vi "scaleEncoder.vi"(8 "error in (no error)":errorcluster, 11 "String":string) -> (0 "error out":errorcluster, 2 "Encoder1":i32, 3 "Encoder0":i32)   [LabVIEW 2017]
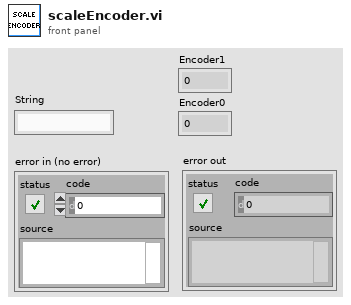
[diagram p1: front panel]
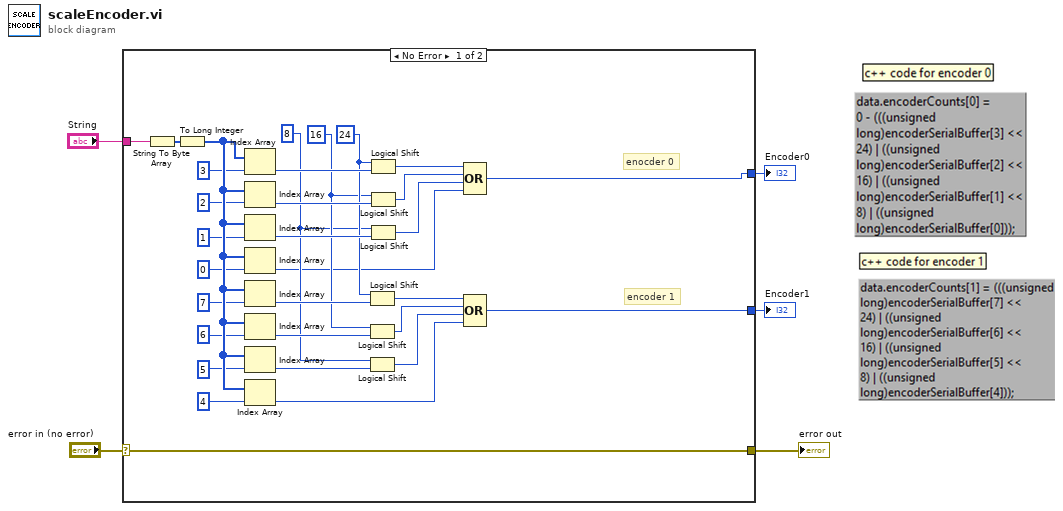
[diagram p0: block diagram]
diagram:
  n1 = case shown="No Error" "error in (no error)" {
    selector: "error in (no error)" -> [w25 w37]
    tunnel: "String" -> [w36 _]
    tunnel: [w25 w37] -> w3
    tunnel: [w7 _] -> w2
    tunnel: [w6 _] -> w1
    frame No Error {
      w16 = 8
      w17 = 16
      w18 = 24
      # "encoder 1"
      # "enocder 0"
      n2 = String To Byte Array(string=w36) -> (unsigned byte array=w35:u8[])
      n3 = To Long Integer(number=w35) -> (32bit integer=w34:i32[])
      n4 = Index Array(array=w34, index=3) -> (element=w24:i32)
      n5 = Index Array(array=w34, index=2) -> (element=w23:i32)
      n6 = Index Array(array=w34, index=1) -> (element=w22:i32)
      n7 = Index Array(array=w34, index=0) -> (element=w12:i32)
      n8 = Index Array(array=w34, index=7) -> (element=w21:i32)
      n9 = Index Array(array=w34, index=6) -> (element=w20:i32)
      n10 = Index Array(array=w34, index=5) -> (element=w19:i32)
      n11 = Index Array(array=w34, index=4) -> (element=w8:i32)
      n12 = Logical Shift(y=w18, x=w21) -> (x << y=w11:i32)
      n13 = Logical Shift(y=w17, x=w20) -> (x << y=w10:i32)
      n14 = Logical Shift(y=w16, x=w19) -> (x << y=w9:i32)
      n15 = Logical Shift(y=w18, x=w24) -> (x << y=w15:i32)
      n16 = Logical Shift(y=w17, x=w23) -> (x << y=w14:i32)
      n17 = Logical Shift(y=w16, x=w22) -> (x << y=w13:i32)
      n18 = Compound Arithmetic op=OR(w15, w14, w13, w12) -> (w6:i32)
      n19 = Compound Arithmetic op=OR(w11, w10, w9, w8) -> (w7:i32)
    }
    frame Error {
    }
  }
  "error out" <- w3
  "Encoder1" <- w2
  "Encoder0" <- w1
